vi "Value Limiter.vi"(1 "Max Limit":i16, 2 "Value":i16) -> (0 "Limited value":i16)   [LabVIEW 2023]
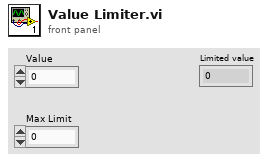
[diagram p1: front panel]
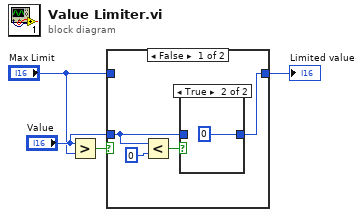
[diagram p0: block diagram]
diagram:
  n1 = Greater?(x="Value", y="Max Limit") -> (0:w4:bool)
  n2 = case shown="False" w4 {
    tunnel: [w6 w11] -> w3
    tunnel: "Value" -> [w5 _]
    tunnel: "Max Limit" -> [_ w11]
    frame False {
      n3 = Less?(x=w5, y=i16 0) -> (x < y?=w8:bool)
      n4 = case shown="True" w8 {
        tunnel: [w9 i16 0 ("Numeric")] -> w6
        tunnel: w5 -> [w9 _]
        frame False {
        }
        frame True {
        }
      }
    }
    frame True {
    }
  }
  "Limited value" <- w3
